vi "Init_timestep_new.vi"(8 "Variables":T2=[{"Value"=10.0, "Variable"="dummy", "Save with Image"=FALSE}, {"Value"=-0.0001, "Variable"="HI", "Save with Image"=FALSE}, {"Value"=-0.0002, "Variable"="LO", "Save with Image"=FALSE}, {"Value"=0.0, "Variable"="dummy1", "Save with Image"=FALSE}, {"Value"=0.0, "Variable"="dummy2", "Save with Image"=FALSE}, {"Value"=0.0, "Variable"="dummy3", "Save with Image"=FALSE}, {"Value"=0.0, "Variable"="tLEDuv", "Save with Image"=FALSE}, {"Value"=1000.0, "Variable"="tMOT0", "Save with Image"=FALSE}, {"Value"=20.0, "Variable"="tMOT1", "Save with Image"=FALSE}, {"Value"=40.0, "Variable"="tMOT2", "Save with Image"=FALSE}, {"Value"=50.0, "Variable"="tMOT3", "Save with Image"=FALSE}, {"Value"=13.0, "Variable"="tMOT3delayREP", "Save with Image"=FALSE}, {"Value"=0.05, "Variable"="tREP", "Save with Image"=FALSE}, {"Value"=0.75, "Variable"="dMOT0", "Save with Image"=FALSE}, {"Value"=1.75, "Variable"="dMOT1", "Save with Image"=FALSE}, {"Value"=1.75, "Variable"="dMOT2", "Save with Image"=FALSE}, {"Value"=0.0, "Variable"="dummy5", "Save with Image"=FALSE}, {"Value"=1.45, "Variable"="pMOT0", "Save with Image"=FALSE}, {"Value"=1.45, "Variable"="pMOT1", "Save with Image"=FALSE}, {"Value"=1.25, "Variable"="pMOT2", "Save with Image"=FALSE}, {"Value"=-1.0, "Variable"="dummy6", "Save with Image"=FALSE}, {"Value"=1.6, "Variable"="pRP0", "Save with Image"=FALSE}, {"Value"=1.6, "Variable"="pRP1", "Save with Image"=FALSE}, {"Value"=0.8, "Variable"="pRP2", "Save with Image"=FALSE}, {"Value"=0.0, "Variable"="MOTdummy0", "Save with Image"=FALSE}, {"Value"=-1.0, "Variable"="MOTdummy1", "Save with Image"=FALSE}, {"Value"=0.0, "Variable"="MOTdummy2", "Save with Image"=FALSE}, {"Value"=0.0, "Variable"="MOTdummy3", "Save with Image"=FALSE}, {"Value"=0.0, "Variable"="MOTdummy4", "Save with Image"=FALSE}, {"Value"=1.8, "Variable"="pCROSS0", "Save with Image"=FALSE}, {"Value"=1.29, "Variable"="pCROSS1", "Save with Image"=FALSE}, {"Value"=1.05, "Variable"="pCROSS2", "Save with Image"=FALSE}, {"Value"=0.75, "Variable"="pCROSS3", "Save with Image"=FALSE}, {"Value"=0.0, "Variable"="pCROSS4", "Save with Image"=FALSE}, {"Value"=5.0, "Variable"="pDIMPL0", "Save with Image"=FALSE}, {"Value"=4.4, "Variable"="pDIMPL1", "Save with Image"=FALSE}, {"Value"=3.65, "Variable"="pDIMPL2", "Save with Image"=FALSE}, {"Value"=3.55, "Variable"="pDIMPL3", "Save with Image"=FALSE}, {"Value"=3.45, "Variable"="pDIMPL4", "Save with Image"=FALSE}, {"Value"=1.8, "Variable"="pTightTrap", "Save with Image"=FALSE}, {"Value"=400.0, "Variable"="tHOLD", "Save with Image"=FALSE}, {"Value"=740.0, "Variable"="tEVAP1", "Save with Image"=FALSE}, {"Value"=2900.0, "Variable"="tEVAP2", "Save with Image"=FALSE}, {"Value"=590.0, "Variable"="tEVAP3", "Save with Image"=FALSE}, {"Value"=50.0, "Variable"="tEVAP4", "Save with Image"=FALSE}, {"Value"=50.0, "Variable"="tHOLDTight", "Save with Image"=FALSE}, {"Value"=0.0, "Variable"="ODTdummy1", "Save with Image"=FALSE}, {"Value"=0.0, "Variable"="ODTdummy2", "Save with Image"=FALSE}, {"Value"=0.0, "Variable"="ODTdummy3", "Save with Image"=FALSE}, {"Value"=0.0, "Variable"="ODTdummy4", "Save with Image"=FALSE}, {"Value"=0.0, "Variable"="ODTdummy5", "Save with Image"=FALSE}, {"Value"=3.59, "Variable"="dIMGx", "Save with Image"=FALSE}, {"Value"=3.59, "Variable"="dIMGx0", "Save with Image"=FALSE}, {"Value"=1.38, "Variable"="dIMGz", "Save with Image"=FALSE}, {"Value"=1.98, "Variable"="dEXCz", "Save with Image"=FALSE}, {"Value"=3.0, "Variable"="pABSx", "Save with Image"=FALSE}, {"Value"=1.35, "Variable"="pABSz", "Save with Image"=FALSE}, {"Value"=0.55, "Variable"="pEXCz", "Save with Image"=FALSE}, {"Value"=0.0, "Variable"="TOF", "Save with Image"=FALSE}, {"Value"=10.0, "Variable"="TOFatomFall", "Save with Image"=FALSE}, {"Value"=0.012, "Variable"="tEXP", "Save with Image"=FALSE}, {"Value"=0.2, "Variable"="tEXP2", "Save with Image"=FALSE}, {"Value"=0.082, "Variable"="tEXC", "Save with Image"=FALSE}, {"Value"=0.001, "Variable"="tWaitIoniz", "Save with Image"=FALSE}, {"Value"=0.065, "Variable"="tCAM", "Save with Image"=FALSE}, {"Value"=200.0, "Variable"="tCAMguppy", "Save with Image"=FALSE}, {"Value"=50.0, "Variable"="tCAMreadout", "Save with Image"=FALSE}, {"Value"=-0.002, "Variable"="tTrigDelay", "Save with Image"=FALSE}, {"Value"=0.0, "Variable"="tTrans", "Save with Image"=FALSE}, {"Value"=1.0, "Variable"="tEXCres", "Save with Image"=FALSE}, {"Value"=0.004, "Variable"="tPUMP", "Save with Image"=FALSE}, {"Value"=2.0, "Variable"="pBLUEswitch", "Save with Image"=FALSE}, {"Value"=2.0, "Variable"="pBLUEswitchEIT", "Save with Image"=FALSE}, {"Value"=3.5, "Variable"="dBLUE", "Save with Image"=FALSE}, {"Value"=3.5, "Variable"="dBLUE0", "Save with Image"=FALSE}, {"Value"=1.7, "Variable"="dBLUEdec", "Save with Image"=FALSE}, {"Value"=2.5, "Variable"="dBLUEdec0", "Save with Image"=FALSE}, {"Value"=3.2, "Variable"="dIMPnew", "Save with Image"=FALSE}, {"Value"=1.0, "Variable"="blueON1", "Save with Image"=FALSE}, {"Value"=0.0, "Variable"="blueON2", "Save with Image"=FALSE}, {"Value"=1.0, "Variable"="blueEXCON1", "Save with Image"=FALSE}, {"Value"=0.0, "Variable"="blueEXCON2", "Save with Image"=FALSE}, {"Value"=35.637858, "Variable"="dRydMW", "Save with Image"=FALSE}, {"Value"=16.0, "Variable"="pRydMW", "Save with Image"=FALSE}, {"Value"=50.0, "Variable"="MWduration", "Save with Image"=FALSE}, {"Value"=4.33, "Variable"="bmw0", "Save with Image"=FALSE}, {"Value"=0.02, "Variable"="bmw1", "Save with Image"=FALSE}, {"Value"=0.0, "Variable"="MWdummy1", "Save with Image"=FALSE}, {"Value"=0.0, "Variable"="MWdummy2", "Save with Image"=FALSE}, {"Value"=0.0, "Variable"="MWdummy3", "Save with Image"=FALSE}, {"Value"=4.3, "Variable"="foffset", "Save with Image"=FALSE}, {"Value"=8.64, "Variable"="fdx", "Save with Image"=FALSE}, {"Value"=-5.78, "Variable"="fdy", "Save with Image"=FALSE}, {"Value"=4.0, "Variable"="fdz", "Save with Image"=FALSE}, {"Value"=300.0, "Variable"="CH203", "Save with Image"=FALSE}, {"Value"=160.0, "Variable"="CH215", "Save with Image"=FALSE}, {"Value"=4.0, "Variable"="CH302", "Save with Image"=FALSE}, {"Value"=280.0, "Variable"="CH315", "Save with Image"=FALSE}, {"Value"=0.0, "Variable"="CH202", "Save with Image"=FALSE}, {"Value"=0.0, "Variable"="CH308", "Save with Image"=FALSE}, {"Value"=0.0, "Variable"="EFIELDdummy2", "Save with Image"=FALSE}, {"Value"=0.0, "Variable"="EFIELDdummy3", "Save with Image"=FALSE}, {"Value"=0.0, "Variable"="EFIELDdummy4", "Save with Image"=FALSE}, {"Value"=0.0, "Variable"="EFIELDdummy5", "Save with Image"=FALSE}, {"Value"=0.0, "Variable"="EFIELDdummy6", "Save with Image"=FALSE}, {"Value"=0.0, "Variable"="EFIELDdummy7", "Save with Image"=FALSE}, {"Value"=1.25, "Variable"="bMOT0", "Save with Image"=FALSE}, {"Value"=2.5, "Variable"="bMOT1", "Save with Image"=FALSE}, {"Value"=2.5, "Variable"="bMOT2", "Save with Image"=FALSE}, {"Value"=1.25, "Variable"="bMOT3", "Save with Image"=FALSE}, {"Value"=0.0, "Variable"="bCOMPx", "Save with Image"=FALSE}, {"Value"=1.35, "Variable"="bCOMPy", "Save with Image"=FALSE}, {"Value"=0.27, "Variable"="bCOMPz", "Save with Image"=FALSE}, {"Value"=0.7, "Variable"="bCOMPx1", "Save with Image"=FALSE}, {"Value"=1.1, "Variable"="bCOMPy1", "Save with Image"=FALSE}, {"Value"=0.5, "Variable"="bCOMPz1", "Save with Image"=FALSE}, {"Value"=4.35, "Variable"="bxfinal", "Save with Image"=FALSE}, {"Value"=0.0, "Variable"="byfinal", "Save with Image"=FALSE}, {"Value"=0.0, "Variable"="bzfinal", "Save with Image"=FALSE}, {"Value"=0.0, "Variable"="BFIELDdummy1", "Save with Image"=FALSE}, {"Value"=0.0, "Variable"="BFIELDdummy2", "Save with Image"=FALSE}, {"Value"=0.0, "Variable"="BFIELDdummy3", "Save with Image"=FALSE}, {"Value"=10.0, "Variable"="tCOILsettle", "Save with Image"=FALSE}, {"Value"=0.0, "Variable"="tRemove", "Save with Image"=FALSE}, {"Value"=3.6, "Variable"="pRemove", "Save with Image"=FALSE}, {"Value"=3.1, "Variable"="dF2CLEAN1x", "Save with Image"=FALSE}, {"Value"=20.0, "Variable"="tF2CLEAN1x", "Save with Image"=FALSE}, {"Value"=4.0, "Variable"="tF2CLEAN2x", "Save with Image"=FALSE}, {"Value"=0.0, "Variable"="tDelayDown", "Save with Image"=FALSE}, {"Value"=156.0, "Variable"="oDDSbluePro", "Save with Image"=FALSE}, {"Value"=-10.25, "Variable"="dDDSbluePro", "Save with Image"=FALSE}, {"Value"=50.0, "Variable"="tRampDDSbluePro", "Save with Image"=FALSE}, {"Value"=416.6261, "Variable"="oDDSred", "Save with Image"=FALSE}, {"Value"=-50.25, "Variable"="dDDSred", "Save with Image"=FALSE}, {"Value"=90.0, "Variable"="tRampDDSred", "Save with Image"=FALSE}, {"Value"=154.0, "Variable"="oDDSblueOld", "Save with Image"=FALSE}, {"Value"=10.0, "Variable"="dDDSblueOld", "Save with Image"=FALSE}, {"Value"=100.0, "Variable"="tRampDDSblueOld", "Save with Image"=FALSE}, {"Value"=1.0, "Variable"="mwON", "Save with Image"=FALSE}, {"Value"=9.4e-05, "Variable"="tRabi", "Save with Image"=FALSE}, {"Value"=9.4e-05, "Variable"="tRabi2", "Save with Image"=FALSE}, {"Value"=5e-05, "Variable"="tRamsey", "Save with Image"=FALSE}, {"Value"=0.0, "Variable"="tRamsey2", "Save with Image"=FALSE}, {"Value"=0.0, "Variable"="tDDSa", "Save with Image"=FALSE}, {"Value"=0.0, "Variable"="tDDSb", "Save with Image"=FALSE}, {"Value"=399.942, "Variable"="dDDSa", "Save with Image"=FALSE}, {"Value"=399.942, "Variable"="dDDSa2", "Save with Image"=FALSE}, {"Value"=0.2, "Variable"="pDDSa", "Save with Image"=FALSE}, {"Value"=1e-07, "Variable"="pDDSa2", "Save with Image"=FALSE}, {"Value"=0.0, "Variable"="phiDDSa", "Save with Image"=FALSE}, {"Value"=0.875, "Variable"="phiDDSa2", "Save with Image"=FALSE}, {"Value"=399.942, "Variable"="dDDSb", "Save with Image"=FALSE}, {"Value"=400.009, "Variable"="dDDSb2", "Save with Image"=FALSE}, {"Value"=0.25, "Variable"="pDDSb", "Save with Image"=FALSE}, {"Value"=1e-07, "Variable"="pDDSb2", "Save with Image"=FALSE}, {"Value"=0.25, "Variable"="phiDDSb", "Save with Image"=FALSE}, {"Value"=0.55, "Variable"="phiDDSb2", "Save with Image"=FALSE}, {"Value"=300.0, "Variable"="tDipole", "Save with Image"=FALSE}, {"Value"=0.7, "Variable"="bCOMPx2", "Save with Image"=FALSE}, {"Value"=0.8, "Variable"="bCOMPy2", "Save with Image"=FALSE}, {"Value"=0.6, "Variable"="bCOMPz2", "Save with Image"=FALSE}, {"Value"=20.0, "Variable"="dMOTRamp1", "Save with Image"=FALSE}, {"Value"=18.0, "Variable"="DMOTload", "Save with Image"=FALSE}, {"Value"=50.0, "Variable"="dMOTRamp2", "Save with Image"=FALSE}, {"Value"=272.0, "Variable"="DMOTimag", "Save with Image"=FALSE}, {"Value"=1000.0, "Variable"="oDDShyperfine", "Save with Image"=FALSE}, {"Value"=0.1, "Variable"="dDDShyperfine", "Save with Image"=FALSE}, {"Value"=0.0, "Variable"="tof", "Save with Image"=FALSE}, {"Value"=262.5, "Variable"="dOPump", "Save with Image"=FALSE}, {"Value"=4500.0, "Variable"="tRampOPump", "Save with Image"=FALSE}, {"Value"=10.0, "Variable"="tOPump", "Save with Image"=FALSE}, {"Value"=1.5, "Variable"="bCOMPx3", "Save with Image"=FALSE}, {"Value"=0.8, "Variable"="bCOMPy3", "Save with Image"=FALSE}, {"Value"=0.0, "Variable"="bCOMPz3", "Save with Image"=FALSE}, {"Value"=0.0, "Variable"="bCOMPx4", "Save with Image"=FALSE}, {"Value"=0.0, "Variable"="bCOMPy4", "Save with Image"=FALSE}, {"Value"=0.0, "Variable"="bCOMPz4", "Save with Image"=FALSE}, {"Value"=0.0, "Variable"="scan2photRes", "Save with Image"=FALSE}, {"Value"=0.0, "Variable"="tEXCsmallProbe", "Save with Image"=FALSE}, {"Value"=0.082, "Variable"="tEXCBlue", "Save with Image"=FALSE}, {"Value"=0.0015, "Variable"="tDownPump", "Save with Image"=FALSE}, {"Value"=98.75, "Variable"="RF1freq1", "Save with Image"=FALSE}, {"Value"=0.1, "Variable"="RF1freq2", "Save with Image"=FALSE}, {"Value"=98.75, "Variable"="dummya", "Save with Image"=FALSE}, {"Value"=0.1, "Variable"="dummyb", "Save with Image"=FALSE}] {"Value" format="%#.9g"}, 10 "waveform sequence":T1 {"Waveform"."envelope" items=["Square", "Gaussian"]}, 11 "Sampling rate":i64=2000000000) -> (0 "segment amplitude":dbl[](array[numeric])=[0.0, 1e-06, 2.5e-06, 3.5e-06, 4.3e-06], 1 "segment phase":dbl[](array[numeric])=[0.0, 1e-06, 2.5e-06, 3.5e-06, 4.3e-06], 2 "segment frequency":dbl[](array[numeric])=[0.0, 1e-06, 2.5e-06, 3.5e-06, 4.3e-06], 3 "segment duration (int)":i32[](array[numeric])=[2000, 3000, 2000, 1600, 4000])   [LabVIEW 2017]
uses:
  waveform_variables_new.ctl
  Software/Rydberg_Control/TypeDefinition/variables.ctl
panel:
  out "waveform output":T1 {"Waveform"."envelope" items=["Square", "Gaussian"]}
  in  "Plot waveform":bool
  in  "Waveform name":u16(ring) items=["Init X", "WAHUHA", "Readout X", "New waveform..."]
  in  "Save waveform":bool
  out "total subsequences":i32=5
  out "segment duration":dbl[](array[numeric])=[2000.0, 3000.0, 2000.0, 1600.0000000000002, 4000.0]
  out "timestep (int)":i32[](array[numeric])=[0, 2000, 5000, 7000, 8600]
  out "timestep":dbl[](array[numeric])=[2000.0, 5000.0, 7000.0, 8600.0, 12600.0]
  out "timestep (ideal)":dbl[](array[numeric])=[1e-06, 2.4999999999999998e-06, 3.4999999999999995e-06, 4.2999999999999995e-06, 6.299999999999999e-06]
  out "time for waveform":dbl[](array[numeric])=[0.0, 1e-06, 2.5e-06, 3.5e-06, 4.3e-06]
  out "total timestep":i32=12600
  # "No."
  # "freq (MHz)"
  # "phase  (deg)"
  # "amplitude (0-1)"
  # "duration (us)"
  # "envelope"
  # "No."
  # "freq (MHz)"
  # "phase  (deg)"
  # "amplitude (0-1)"
  # "duration (us)"
  # "envelope"
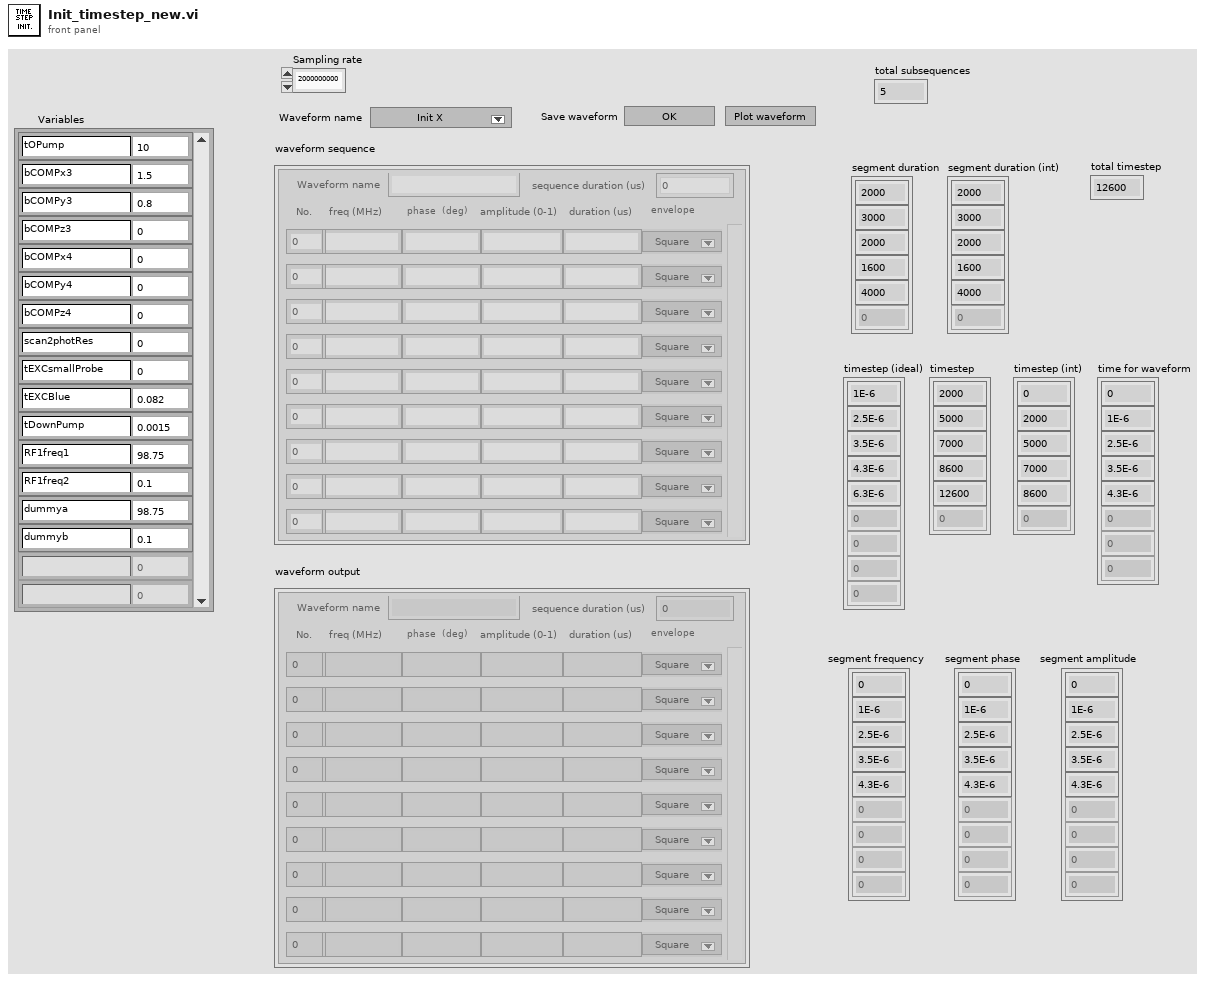
[diagram p1: front panel]
types:
  T1 = typedef "waveform_variables_new.ctl" = cluster{"Waveform name":string, "sequence duration (us)":dbl, "Waveform":cluster{"Segment number":i32, "frequency":string, "phase":string, "amplitude":string, "duration":string, "envelope":u16}[]}[]
  T2 = typedef "variables.ctl" = cluster{"Value":dbl, "Variable":string, "Save with Image":bool}[]
  T3 = cluster{"Waveform name":string, "sequence duration (us)":dbl, "Waveform":cluster{"Segment number":i32, "frequency":string, "phase":string, "amplitude":string, "duration":string, "envelope":u16}[]}
  T4 = cluster{"Segment number":i32, "frequency":string, "phase":string, "amplitude":string, "duration":string, "envelope":u16}[]
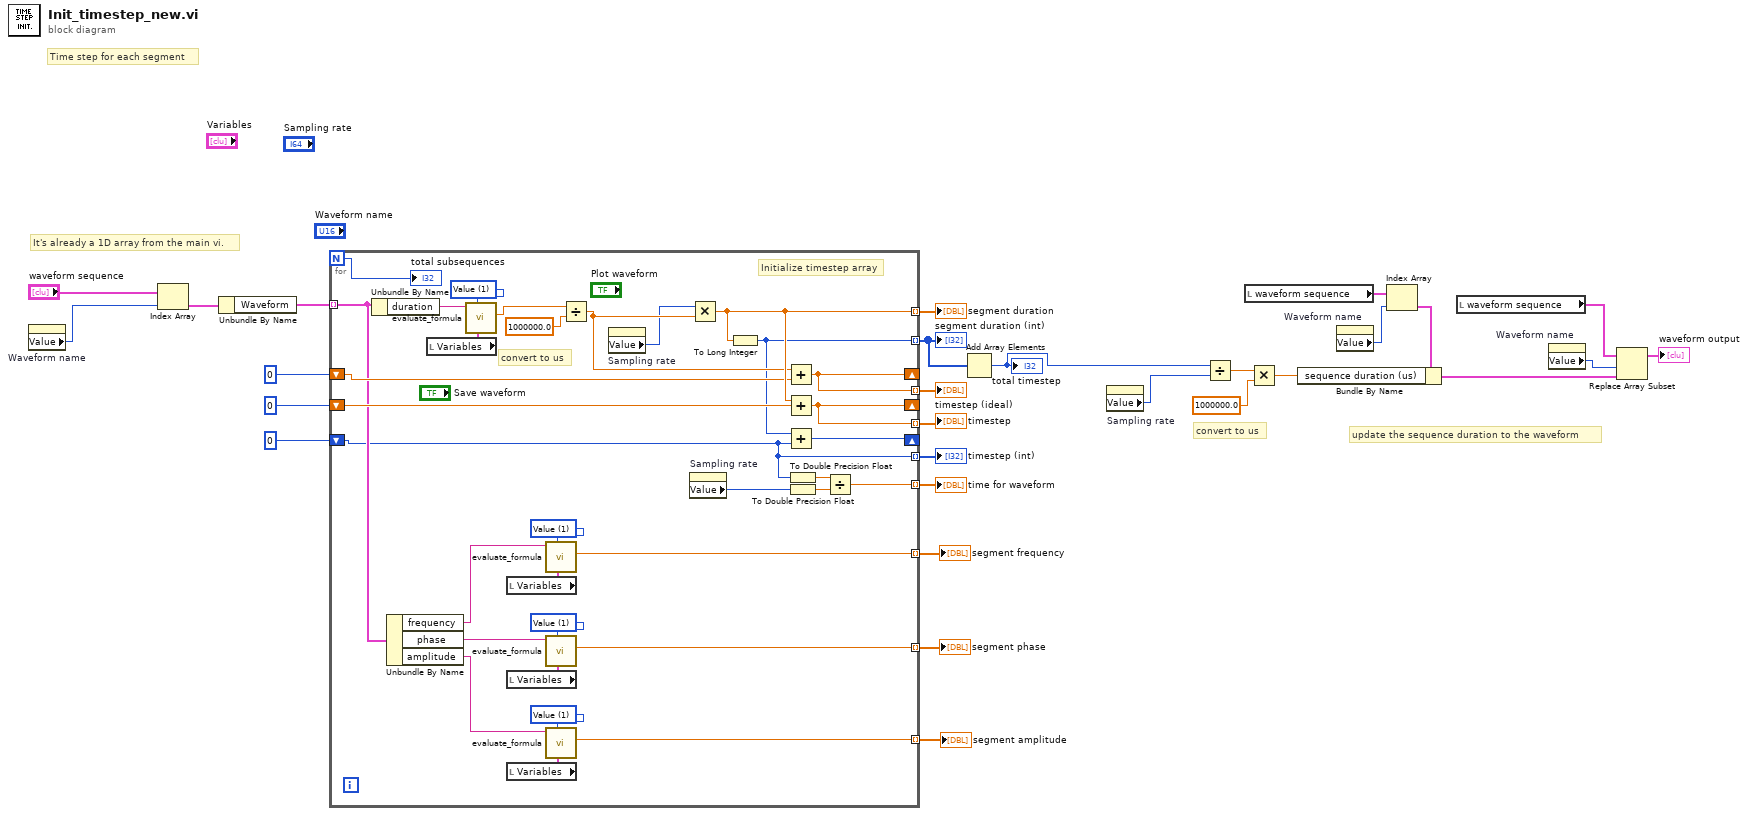
[diagram p0: block diagram]
diagram:
  # "It's already a 1D array from the main vi."
  # "Time step for each segment"
  # "update the sequence duration to the waveform"
  # "convert to us"
  n1 = property on="Waveform name" class="Ring (strict)"() -> ("Value"=w17:u16)  [unwired: 2 in, 2 out]
  n2 = Index Array(array="waveform sequence", index=w17) -> (element=w16:T3)
  n3 = Unbundle By Name(w16) -> ("Waveform"=w28:T4)
  n4 = for {
    N -> [w51]
    tunnel: w28 -> [w45] mode=indexing
    tunnel: [w59] -> w19 mode=indexing
    tunnel: [w52] -> w27 mode=indexing
    shift-right: [w53] -> _
    shift-left: 0 -> [w32]
    tunnel: [w32] -> w21 mode=indexing
    shift-right: [w58] -> _
    shift-left: 0 -> [w60]
    tunnel: [w58] -> w23 mode=indexing
    shift-right: [w55] -> _
    shift-left: 0 -> [w57]
    tunnel: [w55] -> w25 mode=indexing
    tunnel: [w54] -> w26 mode=indexing
    tunnel: [w35] -> w1 mode=indexing
    tunnel: [w34] -> w3 mode=indexing
    tunnel: [w33] -> w2 mode=indexing
    w39 = u16 1 items=["Time in counts", "Value"] ("Time or Value")
    w42 = u16 1 items=["Time in counts", "Value"] ("Time or Value")
    w43 = u16 1 items=["Time in counts", "Value"] ("Time or Value")
    w48 = u16 1 items=["Time in counts", "Value"] ("Time or Value")
    # "Initialize timestep array"
    # "convert to us"
    n5 = Unbundle By Name(w45) -> ("duration"=w47:string)
    n6 = Unbundle By Name(w45) -> ("frequency"=w38:string, "phase"=w37:string, "amplitude"=w36:string)
    n7 = local read "Variables"() -> (w49:T2)
    n8 = call "evaluate_formula.vi"("Variable array"=w49, "Time or Value"=w48, "Formula"=w47) -> ("Output"=w46:dbl)  [unwired: 7 in, 1 out]
    n9 = local read "Variables"() -> (w44:T2)
    n10 = local read "Variables"() -> (w41:T2)
    n11 = local read "Variables"() -> (w40:T2)
    n12 = call "evaluate_formula.vi"("Variable array"=w44, "Time or Value"=w43, "Formula"=w38) -> ("Output"=w35:dbl)  [unwired: 7 in, 1 out]
    n13 = call "evaluate_formula.vi"("Variable array"=w41, "Time or Value"=w42, "Formula"=w37) -> ("Output"=w34:dbl)  [unwired: 7 in, 1 out]
    n14 = call "evaluate_formula.vi"("Variable array"=w40, "Time or Value"=w39, "Formula"=w36) -> ("Output"=w33:dbl)  [unwired: 7 in, 1 out]
    n15 = Divide(x=w46, y=1000000.0) -> (x/y=w56:dbl)
    n16 = property on="Sampling rate" class="DigNum (strict)"() -> ("Value"=w50:i64)  [unwired: 2 in, 2 out]
    n17 = Multiply(x=w50, y=w56) -> (x*y=w59:dbl)
    n18 = property on="Sampling rate" class="DigNum (strict)"() -> ("Value"=w29:i64)  [unwired: 2 in, 2 out]
    n19 = To Long Integer(number=w59) -> (32bit integer=w52:i32)
    n20 = Add(x=w56, y=w57) -> (x+y=w55:dbl)
    n21 = Add(x=w59, y=w60) -> (x+y=w58:dbl)
    n22 = Add(x=w52, y=w32) -> (x+y=w53:i32)
    n23 = To Double Precision Float(number=w32) -> (double precision float=w31:dbl)
    n24 = To Double Precision Float(number=w29) -> (double precision float=w30:dbl)
    n25 = Divide(x=w31, y=w30) -> (x/y=w54:dbl)
    "total subsequences" <- w51
  }
  "segment duration" <- w19
  "segment duration (int)" <- w27
  "timestep (int)" <- w21
  "timestep" <- w23
  "timestep (ideal)" <- w25
  "time for waveform" <- w26
  "segment frequency" <- w1
  "segment phase" <- w3
  "segment amplitude" <- w2
  n26 = Add Array Elements(numeric array=w27) -> (sum=w12:i32)
  "total timestep" <- w12
  n27 = property on="Sampling rate" class="DigNum (strict)"() -> ("Value"=w13:i64)  [unwired: 2 in, 2 out]
  n28 = Divide(x=w12, y=w13) -> (x/y=w14:dbl)
  n29 = local read "waveform sequence"() -> (w7:T1)
  n30 = Multiply(x=w14, y=1000000.0) -> (x*y=w10:dbl)
  n31 = property on="Waveform name" class="Ring (strict)"() -> ("Value"=w8:u16)  [unwired: 2 in, 2 out]
  n32 = Index Array(array=w7, index=w8) -> (element=w11:T3)
  n33 = Bundle By Name(cluster=w11, "sequence duration (us)"=w10) -> (w9:T3)
  n34 = local read "waveform sequence"() -> (w4:T1)
  n35 = property on="Waveform name" class="Ring (strict)"() -> ("Value"=w5:u16)  [unwired: 2 in, 2 out]
  n36 = Replace Array Subset(array=w4, new element=w9, index=w5) -> (→"waveform output":T1)
